vi "Write ImageName.vi"(8 "error in (no error)":errorcluster, 10 "ImageName":string, 11 "Model in":refnum<class "Model.lvclass">) -> (0 "error out":errorcluster, 3 "Model out":refnum<class "Model.lvclass">)   [LabVIEW 2016, in "Model.lvclass"]
uses:
  Model.lvclass
  Model.lvclass/Model.ctl
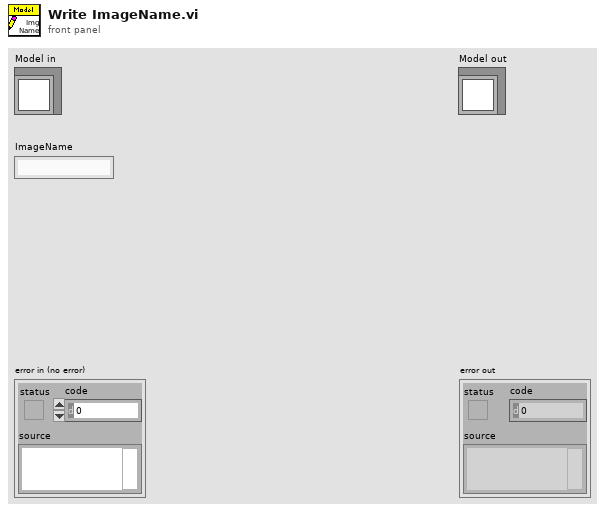
[diagram p1: front panel]
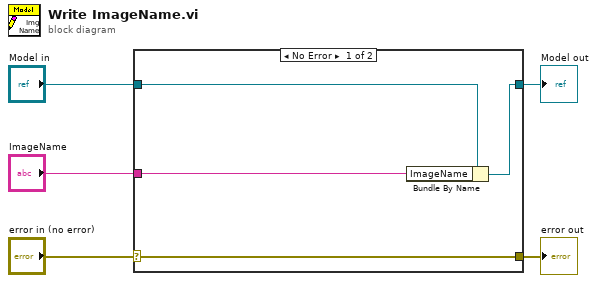
[diagram p0: block diagram]
diagram:
  n1 = case shown="No Error" "error in (no error)" {
    selector: "error in (no error)" -> [w9 w10]
    tunnel: [w9 w10] -> w4
    tunnel: [w7 w11] -> w2
    tunnel: "Model in" -> [w8 w11]
    tunnel: "ImageName" -> [w6 _]
    frame No Error {
      n2 = Bundle By Name(cluster=w8, "ImageName"=w6) -> (w7:refnum<class "Model.lvclass">)
    }
    frame Error {
    }
  }
  "error out" <- w4
  "Model out" <- w2
